vi "SimulateCore.vi"(8 "error in (no error)":errorcluster, 9 "Payload":string, 10 "Command":string, 11 "MicronClient in":refnum<class "MicronClient.lvclass">) -> (0 "error out":errorcluster, 2 "Response":string, 3 "MicronClient out":refnum<class "MicronClient.lvclass">)   [LabVIEW 2019, in "MicronClient.lvclass"]
uses:
  MicronClient.lvclass
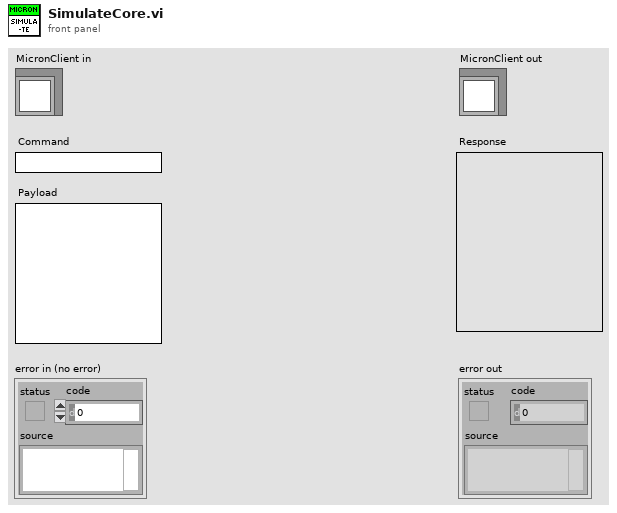
[diagram p1: front panel]
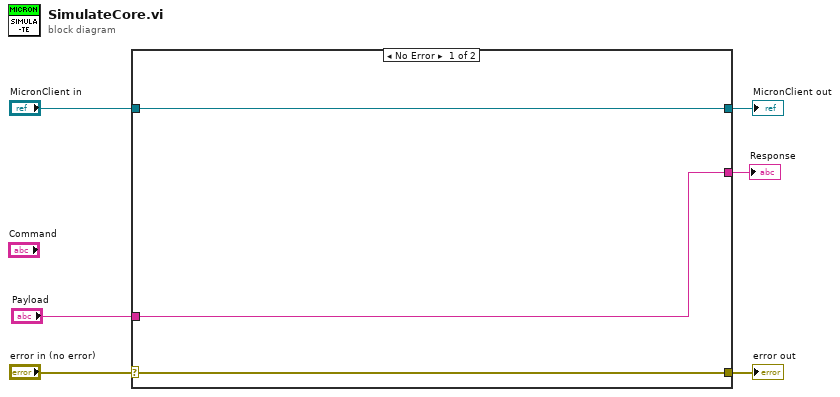
[diagram p0: block diagram]
diagram:
  n1 = case shown="No Error" "error in (no error)" {
    selector: "error in (no error)" -> [w8 w11]
    tunnel: [w8 w11] -> w5
    tunnel: [w9 w10] -> w3
    tunnel: "MicronClient in" -> [w9 w10]
    tunnel: [w7 _] -> w2
    tunnel: "Payload" -> [w7 _]
    frame No Error {
    }
    frame Error {
    }
  }
  "error out" <- w5
  "MicronClient out" <- w3
  "Response" <- w2
